vi "科学计数法转换.vi"() -> ()   [LabVIEW 2014]
panel:
  out "参数显示表 2":string[][](table) caption="Circuit Parameters"
  out "结果字符串":string
  out "电子表格字符串":string
  in  "参数显示表":string[][](table)=[["C_1", "2n"], ["C_2", "20n"], ["L_1", "80u"], ["R_0", "2k"], ["R_1", "2k"], ["R_2", "100"], ["R_3", "8.2k"], ["R_4", "3.3k"], ["R_6", "82k"], ["Rs_1", "10m"], ["Rs_2", "10m"], ["Rv_1", "3.5k"], ["Rv_2", "20k"], ["Load_R_5", "20"], ["Unit_C_3", "1.6m"]] caption="Circuit Parameters"
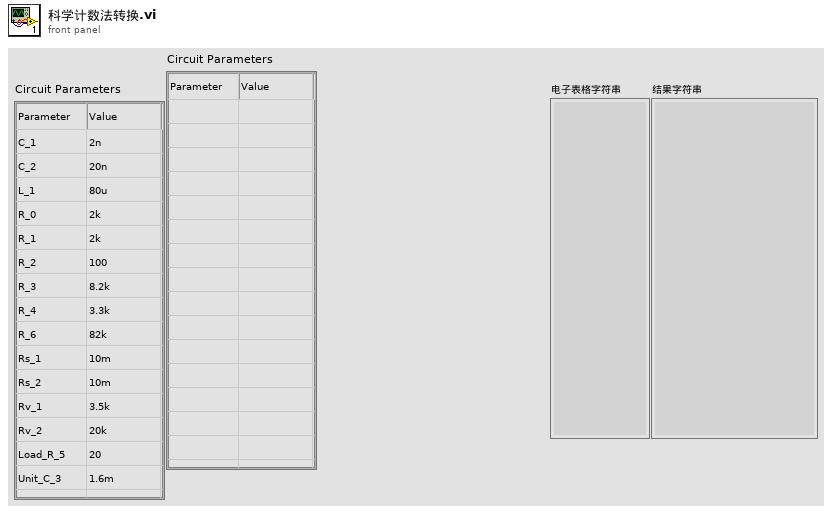
[diagram p1: front panel]
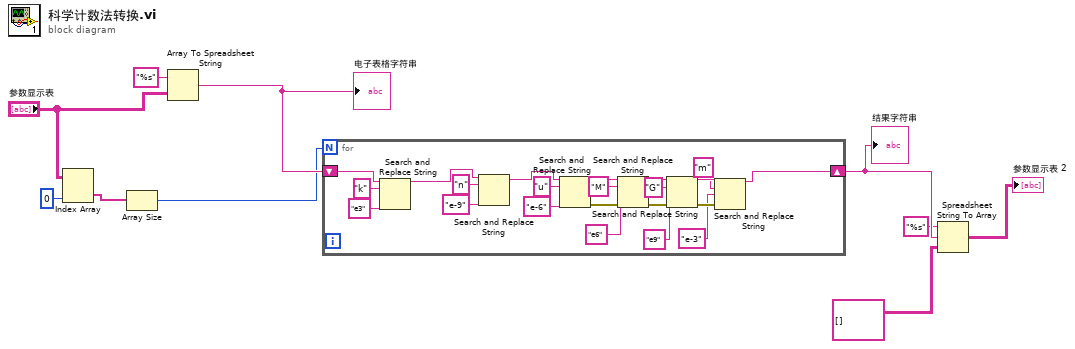
[diagram p0: block diagram]
diagram:
  n1 = Index Array(array="参数显示表", index (col)=0 ("禁用的索引 (列)")) -> (element=w6:string[])  [unwired: 1 in]
  n2 = Array Size(array=w6) -> (size(s)=w5:i32)
  n3 = Array To Spreadsheet String(array="参数显示表", 3:"%s" ("格式字符串")) -> (spreadsheet string=w9:string)  [unwired: 1 in]
  "电子表格字符串" <- w9
  n4 = for {
    N: w5 -> [_]
    shift-right: [w11] -> w4
    shift-left: w9 -> [w30]
    n5 = Search and Replace String(input string=w30, search string="k" ("搜索字符串"), replace string="e3" ("替换字符串(\"\")")) -> (result string=w27:string)  [unwired: 5 in, 3 out]
    n6 = Search and Replace String(input string=w27, search string="n" ("搜索字符串"), replace string="e-9" ("替换字符串(\"\")")) -> (result string=w24:string)  [unwired: 5 in, 3 out]
    n7 = Search and Replace String(input string=w24, search string="u" ("搜索字符串"), replace string="e-6" ("替换字符串(\"\")")) -> (result string=w23:string, error out=w22:errorcluster)  [unwired: 5 in, 2 out]
    n8 = Search and Replace String(input string=w23, search string="M" ("搜索字符串"), replace string="e6" ("替换字符串(\"\")"), error in=w22) -> (result string=w19:string, error out=w18:errorcluster)  [unwired: 4 in, 2 out]
    n9 = Search and Replace String(input string=w19, search string="G" ("搜索字符串"), replace string="e9" ("替换字符串(\"\")"), error in=w18) -> (result string=w15:string, error out=w14:errorcluster)  [unwired: 4 in, 2 out]
    n10 = Search and Replace String(input string=w15, search string="m" ("搜索字符串"), replace string="e-3" ("替换字符串(\"\")"), error in=w14) -> (result string=w11:string)  [unwired: 4 in, 3 out]
  }
  "结果字符串" <- w4
  n11 = Spreadsheet String To Array(format string="%s" ("格式字符串"), spreadsheet string=w4, array type (2D Dbl)=string[][] [] ("Array")) -> (array=→"参数显示表 2":string[][])  [unwired: 1 in]
